vi "fgv_clamp_roi.vi"(7 "cmd":enum16{"init", "read", "write"}(ring), 11 "ROI-clamp":T1) -> (3 "ROI-clamp out":T1)   [LabVIEW 2019]
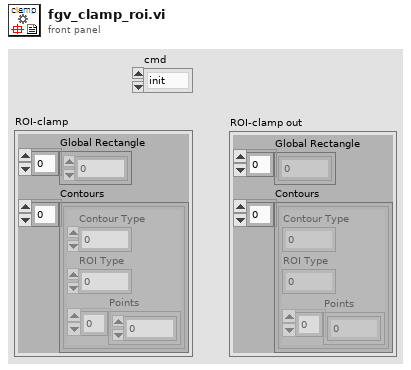
[diagram p1: front panel]
types:
  T1 = cluster{"Global Rectangle":i32[], "Contours":cluster{"Contour Type":u32, "ROI Type":u32, "Points":i32[]}[]}
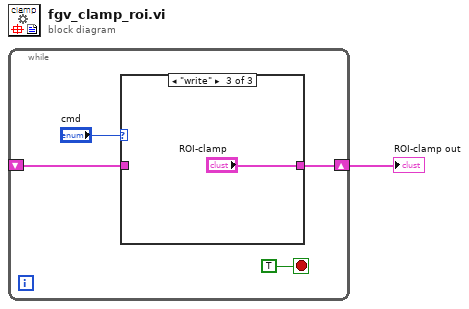
[diagram p0: block diagram]
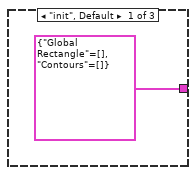
[diagram p2: hidden frame]
diagram:
  n1 = while {
    shift-right: [w3] -> w1
    shift-left: _ -> [w2]
    stop <- TRUE stop-if-true
    n2 = case shown="\"write\"" "cmd" {
      tunnel: [T1 {"Global Rectangle"=[], "Contours"=[]} ("ROI-clamp") w7 "ROI-clamp"] -> w3
      tunnel: w2 -> [_ w7 _]
      frame "init", Default {
      }
      frame "read" {
      }
      frame "write" {
      }
    }
  }
  "ROI-clamp out" <- w1
